vi "XML_CheckExist.vi"(8 "error in (no error)":errorcluster caption="错误输入（无错误）", 10 "label":string="opcua_server", 11 "XML in":T1="<opcua_server><name>server</name><port>4845</port><policy>none</policy><serverCertification></serverCertification><trustedClientCertifications><certification></certification></trustedClientCertifications><structure><folder name=\"all supported datatypes\"><folder name=\"singal element\"><item name=\"boolean\" access=\"read/write\" datatype=\"boolean\" initialValue=\"TRUE\"></item><item name=\"string\" access=\"read/write\" datatype=\"string\" initialValue=\"stringtype\"></item><item name=\"sbyte\" access=\"read/write\" datatype=\"sbyte\" initialValue=\"-10\"></item><item name=\"byte\" access=\"read/write\" datatype=\"byte\" initialValue=\"10\"></item><item name=\"int16\" access=\"read/write\" datatype=\"int16\" initialValue=\"-10\"></item><item name=\"int32\" access=\"read/write\" datatype=\"int32\" initialValue=\"-20\"></item><item name=\"int64\" access=\"read/write\" datatype=\"int64\" initialValue=\"-30\"></item><item name=\"uint16\" access=\"read/write\" datatype=\"uint16\" initialValue=\"10\"></item><item name=\"uint32\" access=\"read/write\" datatype=\"uint32\" initialValue=\"20\"></item><item name=\"uint64\" access=\"read/write\" datatype=\"uint64\" initialValue=\"30\"></item><item name=\"double\" access=\"read/write\" datatype=\"double\" initialValue=\"10.1\"></item><item name=\"float\" access=\"read/write\" datatype=\"float\" initialValue=\"12.1\"></item><item name=\"datetime\" access=\"read/write\" datatype=\"datetime\" initialValue=\"4/30/2004 7:48:47 PM\"></item><item name=\"byte string\" access=\"read/write\" datatype=\"ByteString\" initialValue=\"(1,2,3,4,5)\"></item></folder><folder name=\"array\"><item name=\"boolean array\" access=\"read/write\" datatype=\"boolean array\" initialValue=\"FALSE,TRUE,FALSE\"></item><item name=\"string array\" access=\"read/write\" datatype=\"string array\" initialValue=\"str1,str2,str3\"></item><item name=\"sbyte array\" access=\"read/write\" datatype=\"sbyte array\" initialValue=\"-1,2,-3,4,-5,6,-7,8\"></item><item name=\"byte array\" access=\"read/write\" datatype=\"byte array\" initialValue=\"1,2,3,4,5,6,7,8\"></item><item name=\"int16 array\" access=\"read/write\" datatype=\"int16 array\" initialValue=\"-1,2,-3,4,-5,6,-7,8\"></item><item name=\"int32 array\" access=\"read/write\" datatype=\"int32 array\" initialValue=\"-1,2,-3,4,-5,6,-7,8\"></item><item name=\"int64 array\" access=\"read/write\" datatype=\"int64 array\" initialValue=\"-1,2,-3,4,-5,6,-7,8\"></item><item name=\"uint16 array\" access=\"read/write\" datatype=\"uint16 array\" initialValue=\"1,2,3,4,5,6,7,8\"></item><item name=\"uint32 array\" access=\"read/write\" datatype=\"uint32 array\" initialValue=\"1,2,3,4,5,6,7,8\"></item><item name=\"uint64 array\" access=\"read/write\" datatype=\"uint64 array\" initialValue=\"1,2,3,4,5,6,7,8\"></item><item name=\"double array\" access=\"read/write\" datatype=\"double array\" initialValue=\"1.1,2.2,3.3\"></item><item name=\"float array\" access=\"read/write\" datatype=\"float array\" initialValue=\"1.1,2.2,3.3\"></item><item name=\"datetime array\" access=\"read/write\" datatype=\"datetime array\" initialValue=\"4/30/2004 7:48:47 PM,5/30/2004 8:48:47 PM,6/30/2004 9:48:47 PM\"></item></folder></folder><folder name=\"structure demo\"><folder name=\"device1\"><item name=\"int1\" access=\"read/write\" datatype=\"int32\" initialValue=\"50\" description=\"\"><property name=\"set point\" access=\"read/write\" datatype=\"int32\" initialValue=\"12.4\" description=\"Set point of int1.\"></property><property name=\"status\" access=\"read only\" datatype=\"boolean\" initialValue=\"FALSE\" description=\"Status of int1.\"></property></item></folder><folder name=\"device2\"><folder name=\"device3\"><item name=\"bool1\" access=\"read/write\" datatype=\"boolean\" initialValue=\"FALSE\" description=\"\"><property name=\"set point\" access=\"read/write\" datatype=\"boolean\" initialValue=\"FALSE\" description=\"Set point of bool1.\"></property><property name=\"status\" access=\"read only\" datatype=\"boolean\" initialValue=\"FALSE\" description=\"Status of bool1.\"></property></item></folder><item name=\"str1\" access=\"read/write\" datatype=\"string\" initialValue=\"\" description=\"\"><property name=\"set point\" access=\"read/write\" datatype=\"string\" initialValue=\"test initialize\" description=\"Set point of str1.\"></property><property name=\"status\" access=\"read only\" datatype=\"boolean\" initialValue=\"FALSE\" description=\"Status of str1.\"></property></item></folder><folder name=\"grandpa\"><folder name=\"father\"><folder name=\"son\"><item name=\"son item\" access=\"read/write\" datatype=\"string\" initialValue=\"\" description=\"\"></item></folder></folder></folder><folder name=\"level1\"><folder name=\"level2\"><folder name=\"level3\"><folder name=\"level4\"><folder name=\"level5\"><folder name=\"level6\"><item name=\"data level6\" access=\"read/write\" datatype=\"uint32\" initialValue=\"1000\" description=\"\"></item></folder></folder></folder></folder></folder></folder></folder></structure></opcua_server>") -> (0 "error out":errorcluster caption="错误输出", 1 "exist?":bool, 2 "label (dup)":string="opcua_server", 3 "XML out":T1="<opcua_server><name>server</name><port>4845</port><policy>none</policy><serverCertification></serverCertification><trustedClientCertifications><certification></certification></trustedClientCertifications><structure><folder name=\"all supported datatypes\"><folder name=\"singal element\"><item name=\"boolean\" access=\"read/write\" datatype=\"boolean\" initialValue=\"TRUE\"></item><item name=\"string\" access=\"read/write\" datatype=\"string\" initialValue=\"stringtype\"></item><item name=\"sbyte\" access=\"read/write\" datatype=\"sbyte\" initialValue=\"-10\"></item><item name=\"byte\" access=\"read/write\" datatype=\"byte\" initialValue=\"10\"></item><item name=\"int16\" access=\"read/write\" datatype=\"int16\" initialValue=\"-10\"></item><item name=\"int32\" access=\"read/write\" datatype=\"int32\" initialValue=\"-20\"></item><item name=\"int64\" access=\"read/write\" datatype=\"int64\" initialValue=\"-30\"></item><item name=\"uint16\" access=\"read/write\" datatype=\"uint16\" initialValue=\"10\"></item><item name=\"uint32\" access=\"read/write\" datatype=\"uint32\" initialValue=\"20\"></item><item name=\"uint64\" access=\"read/write\" datatype=\"uint64\" initialValue=\"30\"></item><item name=\"double\" access=\"read/write\" datatype=\"double\" initialValue=\"10.1\"></item><item name=\"float\" access=\"read/write\" datatype=\"float\" initialValue=\"12.1\"></item><item name=\"datetime\" access=\"read/write\" datatype=\"datetime\" initialValue=\"4/30/2004 7:48:47 PM\"></item><item name=\"byte string\" access=\"read/write\" datatype=\"ByteString\" initialValue=\"(1,2,3,4,5)\"></item></folder><folder name=\"array\"><item name=\"boolean array\" access=\"read/write\" datatype=\"boolean array\" initialValue=\"FALSE,TRUE,FALSE\"></item><item name=\"string array\" access=\"read/write\" datatype=\"string array\" initialValue=\"str1,str2,str3\"></item><item name=\"sbyte array\" access=\"read/write\" datatype=\"sbyte array\" initialValue=\"-1,2,-3,4,-5,6,-7,8\"></item><item name=\"byte array\" access=\"read/write\" datatype=\"byte array\" initialValue=\"1,2,3,4,5,6,7,8\"></item><item name=\"int16 array\" access=\"read/write\" datatype=\"int16 array\" initialValue=\"-1,2,-3,4,-5,6,-7,8\"></item><item name=\"int32 array\" access=\"read/write\" datatype=\"int32 array\" initialValue=\"-1,2,-3,4,-5,6,-7,8\"></item><item name=\"int64 array\" access=\"read/write\" datatype=\"int64 array\" initialValue=\"-1,2,-3,4,-5,6,-7,8\"></item><item name=\"uint16 array\" access=\"read/write\" datatype=\"uint16 array\" initialValue=\"1,2,3,4,5,6,7,8\"></item><item name=\"uint32 array\" access=\"read/write\" datatype=\"uint32 array\" initialValue=\"1,2,3,4,5,6,7,8\"></item><item name=\"uint64 array\" access=\"read/write\" datatype=\"uint64 array\" initialValue=\"1,2,3,4,5,6,7,8\"></item><item name=\"double array\" access=\"read/write\" datatype=\"double array\" initialValue=\"1.1,2.2,3.3\"></item><item name=\"float array\" access=\"read/write\" datatype=\"float array\" initialValue=\"1.1,2.2,3.3\"></item><item name=\"datetime array\" access=\"read/write\" datatype=\"datetime array\" initialValue=\"4/30/2004 7:48:47 PM,5/30/2004 8:48:47 PM,6/30/2004 9:48:47 PM\"></item></folder></folder><folder name=\"structure demo\"><folder name=\"device1\"><item name=\"int1\" access=\"read/write\" datatype=\"int32\" initialValue=\"50\" description=\"\"><property name=\"set point\" access=\"read/write\" datatype=\"int32\" initialValue=\"12.4\" description=\"Set point of int1.\"></property><property name=\"status\" access=\"read only\" datatype=\"boolean\" initialValue=\"FALSE\" description=\"Status of int1.\"></property></item></folder><folder name=\"device2\"><folder name=\"device3\"><item name=\"bool1\" access=\"read/write\" datatype=\"boolean\" initialValue=\"FALSE\" description=\"\"><property name=\"set point\" access=\"read/write\" datatype=\"boolean\" initialValue=\"FALSE\" description=\"Set point of bool1.\"></property><property name=\"status\" access=\"read only\" datatype=\"boolean\" initialValue=\"FALSE\" description=\"Status of bool1.\"></property></item></folder><item name=\"str1\" access=\"read/write\" datatype=\"string\" initialValue=\"\" description=\"\"><property name=\"set point\" access=\"read/write\" datatype=\"string\" initialValue=\"test initialize\" description=\"Set point of str1.\"></property><property name=\"status\" access=\"read only\" datatype=\"boolean\" initialValue=\"FALSE\" description=\"Status of str1.\"></property></item></folder><folder name=\"grandpa\"><folder name=\"father\"><folder name=\"son\"><item name=\"son item\" access=\"read/write\" datatype=\"string\" initialValue=\"\" description=\"\"></item></folder></folder></folder><folder name=\"level1\"><folder name=\"level2\"><folder name=\"level3\"><folder name=\"level4\"><folder name=\"level5\"><folder name=\"level6\"><item name=\"data level6\" access=\"read/write\" datatype=\"uint32\" initialValue=\"1000\" description=\"\"></item></folder></folder></folder></folder></folder></folder></folder></structure></opcua_server>")   [LabVIEW 2017]
doc: "Reports whether XML in contains an element with the given label."
uses:
  _XML--String.ctl
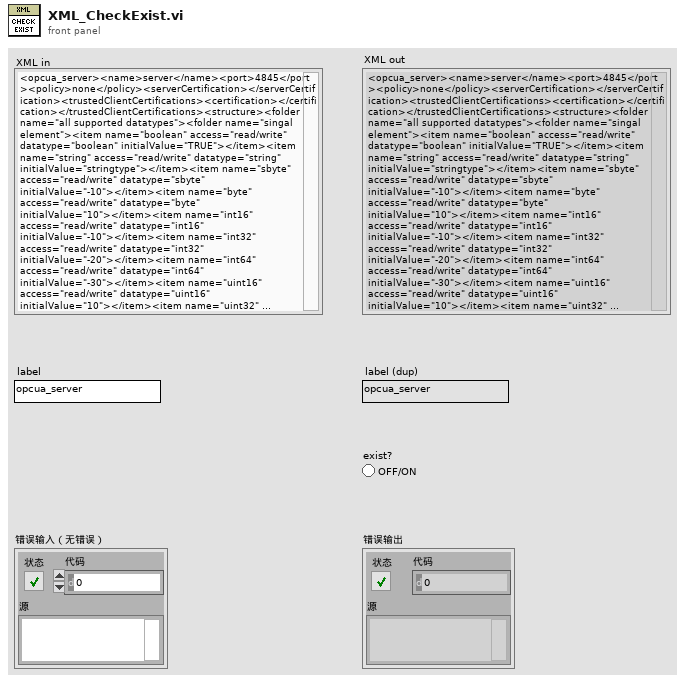
[diagram p1: front panel]
types:
  T1 = typedef "_XML--String.ctl" = string
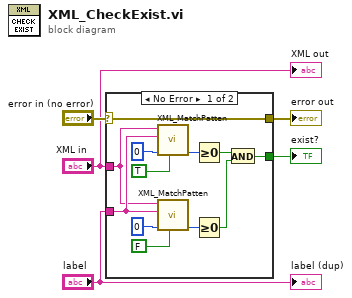
[diagram p0: block diagram]
diagram:
  n1 = case shown="No Error" "error in (no error)" {
    selector: "error in (no error)" -> [w6 w18]
    tunnel: [w6 w18] -> w2
    tunnel: "label" -> [w17 _]
    tunnel: "XML in" -> [w16 _]
    tunnel: [w7 _] -> w1
    frame No Error {
      n2 = call "XML_MatchPatten.vi"("first(T)/Last(F)"=TRUE, "offset (0)"=0, "tag"=w17, "XML"=w16) -> ("offset past match"=w15:i32)  [unwired: 4 in, 3 out]
      n3 = call "XML_MatchPatten.vi"("first(T)/Last(F)"=FALSE, "offset (0)"=0, "tag"=w17, "XML"=w16) -> ("offset past match"=w14:i32)  [unwired: 4 in, 3 out]
      n4 = Greater Or Equal To 0?(x=w15) -> (x >= 0?=w9:bool)
      n5 = Greater Or Equal To 0?(x=w14) -> (x >= 0?=w8:bool)
      n6 = And(x=w9, y=w8) -> (x .and. y?=w7:bool)
    }
    frame Error {
    }
  }
  "error out" <- w2
  "exist?" <- w1
  "XML out" <- "XML in"
  "label (dup)" <- "label"
